vi "LN_GetNodeContent.vi"(3 "InputNode":refnum<class "ListNode.lvclass">) -> (0 "Content":i32, 1 "InputNode 2":refnum<class "ListNode.lvclass">)   [LabVIEW 2014, in "ListNode.lvclass"]
uses:
  ListNode.lvclass
  ListNode.lvclass/ListNode.ctl
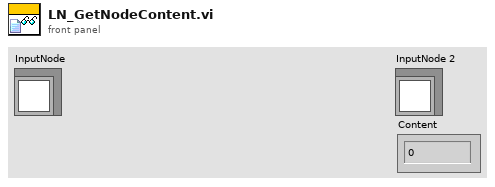
[diagram p1: front panel]
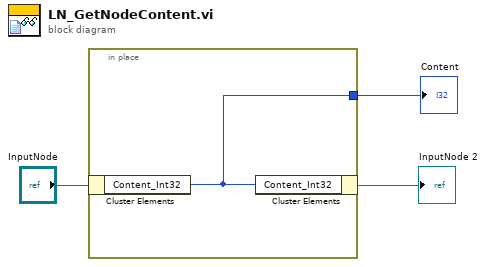
[diagram p0: block diagram]
diagram:
  n1 = in-place {
    in-place-border: [w4] -> w1
    n2 = in-place-cluster #1("InputNode") -> ("Content_Int32"=w4:i32)
    n3 = in-place-cluster #1("Content_Int32"=w4) -> (→"InputNode 2":refnum<class "ListNode.lvclass">)
  }
  "Content" <- w1
